vi "Teleop.vi"(10 "Match Info":T1={"Autonomous Elapsed Seconds"=0.0, "TeleOp Elapsed Seconds"=0.0, "Disabled Elapsed Seconds"=0.0, "Visited Autonomous"=FALSE, "Visited TeleOp"=FALSE, "Visited Disabled"=FALSE, "Autonomous Settings"={"Autonomous Style"=enum."Independent", "VI Refnum"=refnum}}, 11 "Call Context":T2) -> ()   [LabVIEW 2017]
doc: "This VI is called for each enabled TeleOp packet received from the DS. It is typically used to read from joysticks and other inputs and update I/O or setpoints for timed control loops. It should complete and return within 20 milliseconds or risk missing DS packets."
uses:
  <vilib>/Rock Robotics/WPI/DriverStation/WPI_DriverStationDerivedRobotMode.ctl
  <vilib>/Rock Robotics/WPI/DriverStation/WPI_DriverStationMatch Info.ctl
  <vilib>/Rock Robotics/WPI/Utilities/WPI_GetSetVariantRefNum.vi
  <vilib>/Rock Robotics/Network Tables/NT Write Numeric Array.vi
  <vilib>/Rock Robotics/Network Tables/NT Write Boolean Array.vi
  <vilib>/Rock Robotics/WPI/Joystick/WPI_JoystickArcadeMapping.vi
  Drive/Implementation/gyroNumControl.vi
  <vilib>/FRCT Team# 3937  Breakaway/Memory Library/memLib.lvlib
panel:
  out "Steering Graph":cluster{"X":dbl, "Y":dbl}[](graph)
  out "Throttle Graph":cluster{"X":dbl, "Y":dbl}[](graph)
  out "Drive States":cluster{i16, i16, i16, i16, i16}(graph)
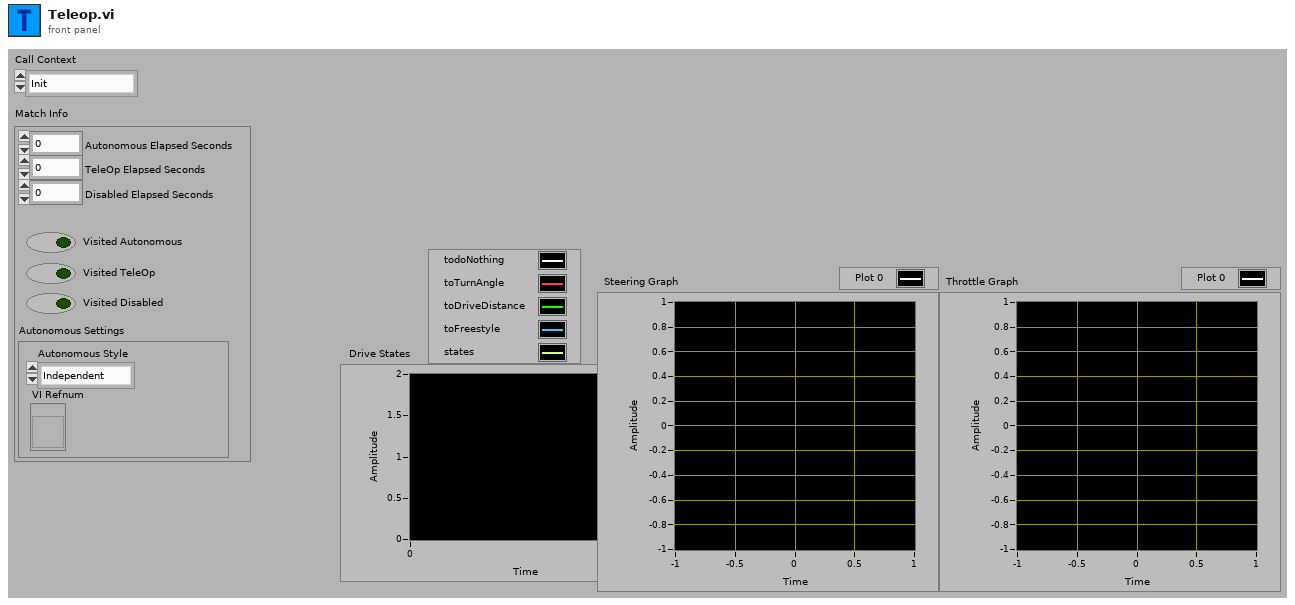
[diagram p1: front panel]
types:
  T1 = typedef "WPI_DriverStationMatch Info.ctl" = cluster{"Autonomous Elapsed Seconds":dbl, "TeleOp Elapsed Seconds":dbl, "Disabled Elapsed Seconds":dbl, "Visited Autonomous":bool, "Visited TeleOp":bool, "Visited Disabled":bool, "Autonomous Settings":cluster{"Autonomous Style":enum16{"Iterative", "Independent"}, "VI Refnum":refnum<vi>}}
  T2 = typedef "WPI_DriverStationDerivedRobotMode.ctl" = enum16{"Init", "Execute", "Stop"}
  T3 = typedef "WPI_JoystickDevRef.ctl" = cluster{"Device":T4}
  T4 = typedef "WPI_JoystickDeviceEnum.ctl" = enum16{"USB 0", "USB 1", "USB 2", "USB 3", "USB 4", "USB 5"}
  T5 = typedef "WPI_SwitchDevRef.ctl" = cluster{"DevStatus":errorcluster, "DIO Channel":T6, "CntIndex":T7, "Normally Closed":bool}
  T6 = typedef "FPGA_DIOChannel.ctl" = enum8{"DIO 0", "DIO 1", "DIO 2", "DIO 3", "DIO 4", "DIO 5", "DIO 6", "DIO 7", "DIO 8", "DIO 9", "DIO MXP 0", "DIO MXP 1", "DIO MXP 2", "DIO MXP 3", "DIO MXP 4", "DIO MXP 5", "DIO MXP 6", "DIO MXP 7", "DIO MXP 8", "DIO MXP 9", "DIO MXP 10", "DIO MXP 11", "DIO MXP 12", "DIO MXP 13", "DIO MXP 14", "DIO MXP 15", "SPI Port CS1", "SPI Port CS2", "SPI Port CS3", "SPI Port MISO", "SPI Port MOSI", "Invalid"}
  T7 = typedef "FPGA_CounterCtrSystemIndex.ctl" = enum8{"Ctr 0", "Ctr 1", "Ctr 2", "Ctr 3", "Ctr 4", "Ctr 5", "Ctr 6", "Ctr 7", "Invalid"}
  T8 = typedef "WPI_MotorControlDeviceRef.ctl" = cluster{"DeviceStatus":errorcluster, "Type":T9, "PWM":cluster{"PWM Channel":T10, "DeadBand":T11}, "CAN":cluster{"Device Number":u8, "SetOutput VI Ref":variant, "GetOutput VI Ref":variant, "Enable VI Ref":variant, "Disable VI Ref":variant, "Data":variant}, "Invert":bool, "DIO PWM":cluster{"PWM \"Enable\" Channel":T10, "DIOChannel":T6, "PWM Rate":dbl}}
  T9 = typedef "WPI_MotorControlType.ctl" = enum16{"PWM", "CAN", "DIO PWM"}
  T10 = typedef "FPGA_DIOPWMChannel.ctl" = enum8{"PWM 0", "PWM 1", "PWM 2", "PWM 3", "PWM 4", "PWM 5", "PWM 6", "PWM 7", "PWM 8", "PWM 9", "PWM MXP 0", "PWM MXP 1", "PWM MXP 2", "PWM MXP 3", "PWM MXP 4", "PWM MXP 5", "PWM MXP 6", "PWM MXP 7", "PWM MXP 8", "PWM MXP 9", "Invalid"}
  T11 = typedef "WPI_PWMDeadband.ctl" = cluster{"Name":string, "maxPositivePwm":i32, "minPositivePwm":i32, "centerPwm":i32, "maxNegativePwm":i32, "minNegativePwm":i32, "angularRange":u16}
  T12 = typedef "Drive Operations.ctl" = enum16{"Reserve", "Read Current", "Freestyle", "Drive for Distance", "TurnAngle", "Guided Drive"}
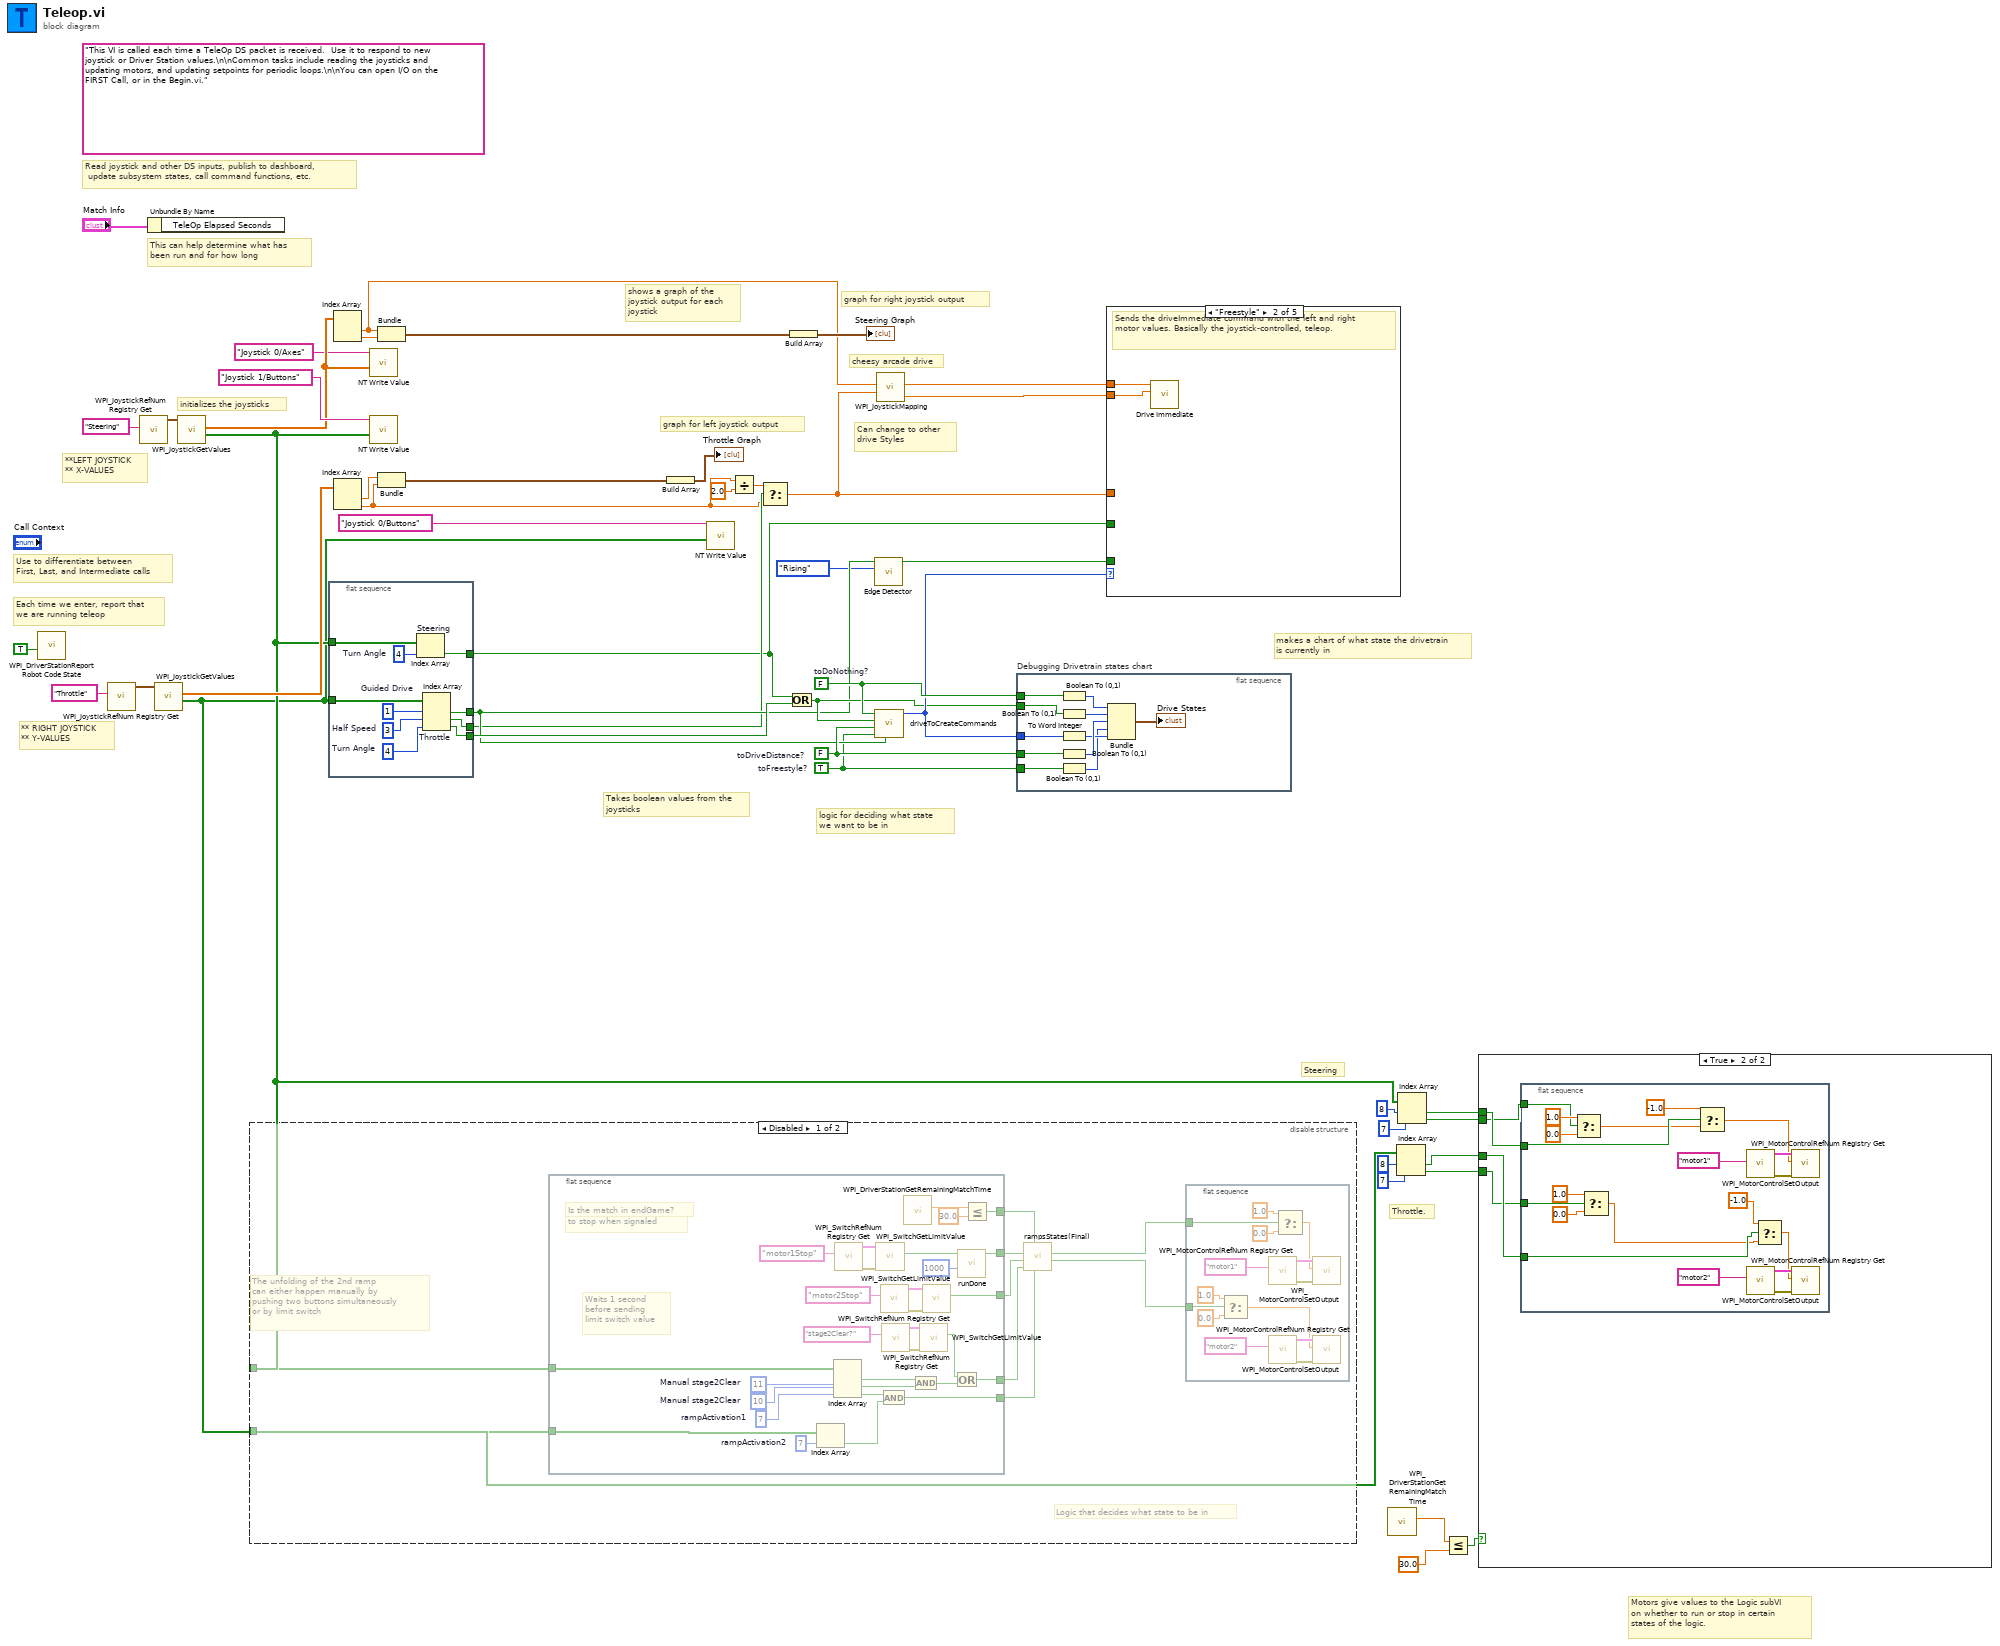
[diagram p0: block diagram]
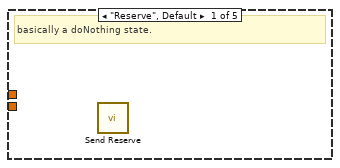
[diagram p4: hidden frame]
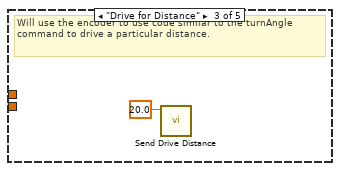
[diagram p5: hidden frame]
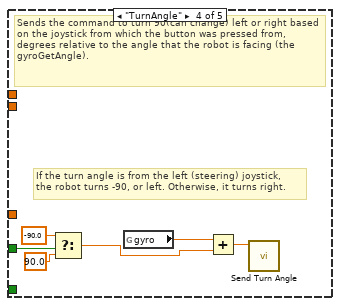
[diagram p6: hidden frame]
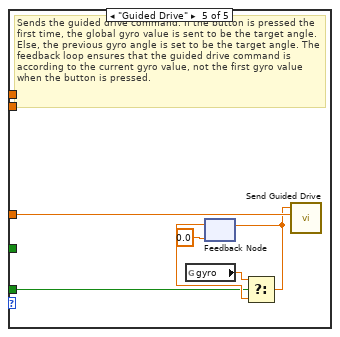
[diagram p7: hidden frame]
diagram:
  w15 = TRUE  # toFreestyle?
  w33 = FALSE  # toDriveDistance?
  w32 = FALSE  # toDoNothing?
  (unwired) "This VI is called each time a TeleOp DS packet is received.  Use it to respond to new joystick or Driver Station values.\n\nCommon tasks include reading the joysticks and updating motors, and updating setpoints for periodic loops.\n\nYou can open I/O on the FIRST Call, or in the Begin.vi."
  # "Throttle."
  # "Steering"
  # "Motors give values to the Logic subVI\non whether to run or stop in certain \nstates of the logic."
  # "Takes boolean values from the\njoysticks"
  # "**LEFT JOYSTICK\n** X-VALUES"
  # "** RIGHT JOYSTICK\n** Y-VALUES"
  # "graph for left joystick output"
  # "graph for right joystick output"
  # "Can change to other\ndrive Styles"
  # "logic for deciding what state\nwe want to be in"
  # "cheesy arcade drive"
  # "makes a chart of what state the drivetrain\nis currently in"
  # "shows a graph of the\njoystick output for each\njoystick"
  # "initializes the joysticks"
  # "Read joystick and other DS inputs, publish to dashboard,\n update subsystem states, call command functions, etc."
  # "Each time we enter, report that\nwe are running teleop"
  # "Use to differentiate between\nFirst, Last, and Intermediate calls"
  # "This can help determine what has\nbeen run and for how long"
  n1 = call <vilib>:"WPI_DriverStationReport Robot Code State.vi"("TeleOp"=TRUE ("Autonomous")) -> ()  [unwired: 10 in, 1 out]
  n2 = call <vilib>:"WPI_JoystickRefNum Registry Get.vi"("refnum name"="Throttle") -> ("JoystickDevRef"=w26:T3)  [unwired: 1 in, 9 out]
  n3 = call <vilib>:"WPI_JoystickRefNum Registry Get.vi"("refnum name"="Steering") -> ("JoystickDevRef"=w25:T3)  [unwired: 1 in, 9 out]
  n4 = Unbundle By Name("Match Info") -> ()  [unwired: 1 out]
  n5 = call <vilib>:"WPI_JoystickGetValues.vi"("JoystickDevRef"=w26) -> ("Buttons"=w12:bool[], "Axes"=w41:dbl[])  [unwired: 6 in, 3 out]
  n6 = call <vilib>:"WPI_JoystickGetValues.vi"("JoystickDevRef"=w25) -> ("Buttons"=w13:bool[], "Axes"=w44:dbl[])  [unwired: 6 in, 3 out]
  n7 = disable-structure shown="Disabled" {
    disable-tunnel: w13 -> [w57 _]
    disable-tunnel: w12 -> [w56 _]
    frame Disabled {
      # "Logic that decides what state to be in"
      # "The unfolding of the 2nd ramp\ncan either happen manually by \npushing two buttons simultaneously\nor by limit switch"
      n8 = flat-sequence {
        tunnel: [w75] -> w54
        tunnel: [w89] -> w52
        tunnel: [w92] -> w55
        tunnel: w56 -> [w86]
        tunnel: w57 -> [w87]
        tunnel: [w81] -> w53
        tunnel: [w72] -> w51
        frame #0 {
          w80 = 11  # Manual stage2Clear
          w88 = 7  # rampActivation1
          w90 = 7  # rampActivation2
          w91 = 10  # Manual stage2Clear
          # "Waits 1 second\nbefore sending \nlimit switch value"
          # "Limit Switch tells motors\nto stop when signaled"
          # "Is the match in endGame?"
          n9 = Index Array(array=w86, index=w90) -> (element=w73:bool)
          n10 = Index Array(array=w87, index #1=w80, index #2=w91, index #3=w88) -> (element #1=w79:bool, element #2=w85:bool, element #3=w74:bool)
          n11 = call <vilib>:"WPI_SwitchRefNum Registry Get.vi"("refnum name"="motor1Stop") -> ("error out"=w99:errorcluster, "SwitchDevRef"=w100:T5)  [unwired: 9 in]
          n12 = call <vilib>:"WPI_SwitchGetLimitValue.vi"("error in (no error)"=w99, "SwitchDevRef"=w100) -> ("Switch Pressed"=w77:bool)  [unwired: 7 in, 2 out]
          n13 = And(x=w74, y=w73) -> (x .and. y?=w72:bool)
          n14 = call <vilib>:"WPI_SwitchRefNum Registry Get.vi"("refnum name"="motor2Stop") -> ("error out"=w83:errorcluster, "SwitchDevRef"=w84:T5)  [unwired: 9 in]
          n15 = call <vilib>:"WPI_SwitchRefNum Registry Get.vi"("refnum name"="stage2Clear?") -> ("error out"=w97:errorcluster, "SwitchDevRef"=w98:T5)  [unwired: 9 in]
          n16 = call <vilib>:"WPI_DriverStationGetRemainingMatchTime.vi"() -> ("Match Time(s)"=w94:sgl)  [unwired: 10 in, 1 out]
          n17 = And(x=w79, y=w85) -> (x .and. y?=w78:bool)
          n18 = call <vilib>:"WPI_SwitchGetLimitValue.vi"("error in (no error)"=w97, "SwitchDevRef"=w98) -> ("Switch Pressed"=w95:bool)  [unwired: 7 in, 2 out]
          n19 = call <vilib>:"WPI_SwitchGetLimitValue.vi"("error in (no error)"=w83, "SwitchDevRef"=w84) -> ("Switch Pressed"=w81:bool)  [unwired: 7 in, 2 out]
          n20 = Or(x=w95, y=w78) -> (x .or. y?=w89:bool)
          n21 = call "runDone.vi"("desiredTime"=1000, "startTimer"=w77) -> ("doneRunning?"=w75:bool)  [unwired: 9 in]
          n22 = Less Or Equal?(x=w94, y=sgl 30.0 ("Match Time(s)")) -> (x <= y?=w92:bool)
        }
      }
      n23 = call "rampsStates(Final).vi"("buttonsPushed?"=w51, "endGame?"=w55, "stage2Clear?"=w52, "motor2Stop"=w53, "motor1Stop"=w54) -> ("rampMotor"=w49:bool, "platformMotor"=w50:bool)  [unwired: 5 in]
      n24 = flat-sequence {
        tunnel: w50 -> [w59]
        tunnel: w49 -> [w58]
        frame #0 {
          n25 = Select(t=1.0, s=w58, f=0.0) -> (s? t:f=w62:dbl)
          n26 = call <vilib>:"WPI_MotorControlRefNum Registry Get.vi"("refnum name"="motor1") -> ("error out"=w69:errorcluster, "MotorControlDevRef"=w70:T8)  [unwired: 9 in]
          n27 = call <vilib>:"WPI_MotorControlRefNum Registry Get.vi"("refnum name"="motor2") -> ("error out"=w63:errorcluster, "MotorControlDevRef"=w64:T8)  [unwired: 9 in]
          n28 = Select(t=1.0, s=w59, f=0.0) -> (s? t:f=w68:dbl)
          n29 = call <vilib>:"WPI_MotorControlSetOutput.vi"("error in (no error)"=w69, "Output"=w68, "MotorControlDevRef"=w70) -> ()  [unwired: 6 in, 3 out]
          n30 = call <vilib>:"WPI_MotorControlSetOutput.vi"("error in (no error)"=w63, "Output"=w62, "MotorControlDevRef"=w64) -> ()  [unwired: 6 in, 3 out]
        }
      }
    }
    frame Enabled {
    }
  }
  n31 = flat-sequence {
    tunnel: w13 -> [w111]
    tunnel: w12 -> [w105]
    tunnel: [w109] -> w14
    tunnel: [w102] -> w28
    tunnel: [w104] -> w24
    tunnel: [w103] -> w20
    frame #0 {
      w106 = 4  # Turn Angle
      w107 = 3  # Half Speed
      w108 = 1  # Guided Drive
      w110 = 4  # Turn Angle
      n32 = Index Array "Steering"(array=w111, index=w110) -> (element=w109:bool)
      n33 = Index Array "Throttle"(array=w105, index #1=w108, index #2=w107, index #3=w106) -> (element #1=w104:bool, element #2=w103:bool, element #3=w102:bool)
    }
  }
  n34 = Index Array(array=w44) -> (element #1=w21:dbl, element #2=w35:dbl)  [unwired: 2 in]
  n35 = Index Array(array=w41) -> (element #1=w34:dbl, element #2=w18:dbl)  [unwired: 2 in]
  n36 = call-poly <vilib>:"NT Write Value.vi"("Numeric Array"=w44, "Name"="Joystick 0/Axes") -> ()  [unwired: 9 in, 1 out]
  n37 = call-poly <vilib>:"NT Write Value.vi"("Boolean Array"=w13, "Name"="Joystick 1/Buttons") -> ()  [unwired: 9 in, 1 out]
  n38 = Bundle("upper limit"=w21, "upper limit"=w35) -> (w37:cluster{"upper limit":dbl, "upper limit":dbl})  [unwired: 1 in]
  n39 = Bundle("upper limit"=w34, "upper limit"=w18) -> (w39:cluster{"upper limit":dbl, "upper limit":dbl})  [unwired: 1 in]
  n40 = Build Array(w39) -> (→"Throttle Graph":cluster{"upper limit":dbl, "upper limit":dbl}[])
  n41 = call-poly <vilib>:"NT Write Value.vi"("Boolean Array"=w12, "Name"="Joystick 0/Buttons") -> ()  [unwired: 9 in, 1 out]
  n42 = Divide(x=w18, y=2.0) -> (x/y=w17:dbl)
  n43 = Select(t=w17, s=w20, f=w18) -> (s? t:f=w16:dbl)
  n44 = Or(x=w14, y=w28) -> (x .or. y?=w27:bool)
  n45 = Build Array(w37) -> (→"Steering Graph":cluster{"upper limit":dbl, "upper limit":dbl}[])
  n46 = call <vilib>:"Edge Detector.vi"("Mode"=enum16{"Rising", "Falling", "Any"}."Rising", "Input"=w24) -> ("Output"=w22:bool)  [unwired: 9 in]
  n47 = call "driveToCreateCommands.vi"("toGuidedDrive"=w24, "toFreestyle"=w15, "toDriveDistance"=w33, "toTurnAngle"=w27, "toReserve"=w32) -> ("Current State"=w31:T12)  [unwired: 6 in]
  n48 = call-poly <vilib>:"WPI_JoystickMapping.vi"("Y axis value"=w16, "X axis value"=w21) -> ("Right Motor Value"=w29:dbl, "Left Motor Value"=w30:dbl)  [unwired: 8 in]
  n49 = flat-sequence "Debugging Drivetrain states chart" {
    tunnel: w33 -> [w122]
    tunnel: w27 -> [w121]
    tunnel: w32 -> [w120]
    tunnel: w31 -> [w114]
    tunnel: w15 -> [w113]
    frame #0 {
      n50 = Boolean To (0,1)(Boolean=w120) -> (0, 1=w117:i16)
      n51 = Boolean To (0,1)(Boolean=w121) -> (0, 1=w118:i16)
      n52 = To Word Integer(number=w114) -> (16bit integer=w115:i16)
      n53 = Boolean To (0,1)(Boolean=w122) -> (0, 1=w119:i16)
      n54 = Boolean To (0,1)(Boolean=w113) -> (0, 1=w112:i16)
      n55 = Bundle(w117, w118, w119, w112, w115) -> (→"Drive States":cluster{i16, i16, i16, i16, i16})  [unwired: 1 in]
    }
  }
  n56 = case shown="\"Freestyle\"" w31 {
    tunnel: w30 -> [_ w124 _ _ _]
    tunnel: w29 -> [_ w123 _ _ _]
    tunnel: w16 -> [_ _ _ _ w137]
    tunnel: w22 -> [_ _ _ _ w132]
    tunnel: w14 -> [_ _ _ w129 _]
    frame "Reserve", Default {
      # "basically a doNothing state."
      n57 = call "Send Reserve.vi"() -> ()  [unwired: 10 in, 2 out]
    }
    frame "Freestyle" {
      # "Sends the driveImmediate command with the left and right motor values. Basically the joystick-controlled, teleop."
      n58 = call "Drive Immediate.vi"("Right Setpoint"=w123, "Left Setpoint"=w124) -> ()  [unwired: 9 in, 1 out]
    }
    frame "Drive for Distance" {
      # "Will use the encoder to use code similar to the turnAngle command to drive a particular distance."
      n59 = call "Send Drive Distance.vi"("Target Distance"=20.0) -> ()  [unwired: 9 in, 2 out]
    }
    frame "TurnAngle" {
      # "If the turn angle is from the left (steering) joystick, \nthe robot turns -90, or left. Otherwise, it turns right."
      # "Sends the command to turn 90(can change) left or right based on the joystick from which the button was pressed from, degrees relative to the angle that the robot is facing (the gyroGetAngle)."
      n60 = Select(t=-90.0, s=w129, f=90.0) -> (s? t:f=w126:dbl)
      n61 = global read "gyroNumControl.vi" "gyro"() -> (w131:dbl)
      n62 = Add(x=w131, y=w126) -> (x+y=w130:dbl)
      n63 = call "Send Turn Angle.vi"("Target Angle"=w130) -> ()  [unwired: 9 in, 2 out]
    }
    frame "Guided Drive" {
      # "Sends the guided drive command. If the button is pressed the first time, the global gyro value is sent to be the target angle. Else, the previous gyro angle is set to be the target angle. The feedback loop ensures that the guided drive command is according to the current gyro value, not the first gyro value when the button is pressed."
      n64 = global read "gyroNumControl.vi" "gyro"() -> (w133:dbl)
      n65 = feedback #1(0.0 ("Angle")) -> (w134:dbl)
      n66 = Select(t=w133, s=w132, f=w134) -> (s? t:f=w136:dbl)
      n67 = feedback-in #1(w136) -> ()
      n68 = call "Send Guided Drive.vi"("Y-value"=w137, "Target Angle"=w136) -> ()  [unwired: 8 in, 2 out]
    }
  }
  n69 = call <vilib>:"WPI_DriverStationGetRemainingMatchTime.vi"() -> ("Match Time(s)"=w7:sgl)  [unwired: 10 in, 1 out]
  n70 = Index Array(array=w12, index #1=8 ("index"), index #2=7 ("index")) -> (element #1=w3:bool, element #2=w1:bool)
  n71 = Index Array(array=w13, index #1=8 ("index"), index #2=7 ("index")) -> (element #1=w4:bool, element #2=w2:bool)
  n72 = Less Or Equal?(x=w7, y=sgl 30.0 ("Match Time(s)")) -> (x <= y?=w5:bool)
  n73 = case shown="True" w5 {
    tunnel: w4 -> [_ w141]
    tunnel: w3 -> [_ w140]
    tunnel: w2 -> [_ w138]
    tunnel: w1 -> [_ w139]
    frame False {
    }
    frame True {
      n74 = flat-sequence {
        tunnel: w141 -> [w151]
        tunnel: w140 -> [w150]
        tunnel: w139 -> [w149]
        tunnel: w138 -> [w142]
        frame #0 {
          n75 = Select(t=1.0, s=w142, f=0.0) -> (s? t:f=w145:dbl)
          n76 = Select(t=1.0, s=w149, f=0.0) -> (s? t:f=w146:dbl)
          n77 = Select(t=-1.0, s=w151, f=w145) -> (s? t:f=w158:dbl)
          n78 = call <vilib>:"WPI_MotorControlRefNum Registry Get.vi"("refnum name"="motor1") -> ("error out"=w159:errorcluster, "MotorControlDevRef"=w160:T8)  [unwired: 9 in]
          n79 = call <vilib>:"WPI_MotorControlRefNum Registry Get.vi"("refnum name"="motor2") -> ("error out"=w154:errorcluster, "MotorControlDevRef"=w155:T8)  [unwired: 9 in]
          n80 = Select(t=-1.0, s=w150, f=w146) -> (s? t:f=w153:dbl)
          n81 = call <vilib>:"WPI_MotorControlSetOutput.vi"("error in (no error)"=w159, "Output"=w158, "MotorControlDevRef"=w160) -> ()  [unwired: 6 in, 3 out]
          n82 = call <vilib>:"WPI_MotorControlSetOutput.vi"("error in (no error)"=w154, "Output"=w153, "MotorControlDevRef"=w155) -> ()  [unwired: 6 in, 3 out]
        }
      }
    }
  }
